vi "hydraharp_acquire_fast.vi"(8 "error in (no error)":errorcluster, 10 "hydraharp_panel out":refnum<class "hydraharp_panel.lvclass">, 11 "hydraharp in":refnum<class "hydraharp.lvclass">) -> (0 "error out":errorcluster, 3 "hydraharp out":refnum<class "hydraharp.lvclass">)   [LabVIEW 2015, in "hydraharp.lvclass"]
uses:
  hydraharp.lvclass
  record_type.ctl
  hydraharp_panel/hydraharp_panel.lvclass
  hydraharp.lvclass/hydraharp.ctl
  UI/panel_class/panel.lvclass/panel.ctl
  hydraharp_fifo_queue_data.ctl
  hydraharp_fifo_actions.ctl
  UI/panel_class/panel.lvclass
panel:
  out "Log Type":T1
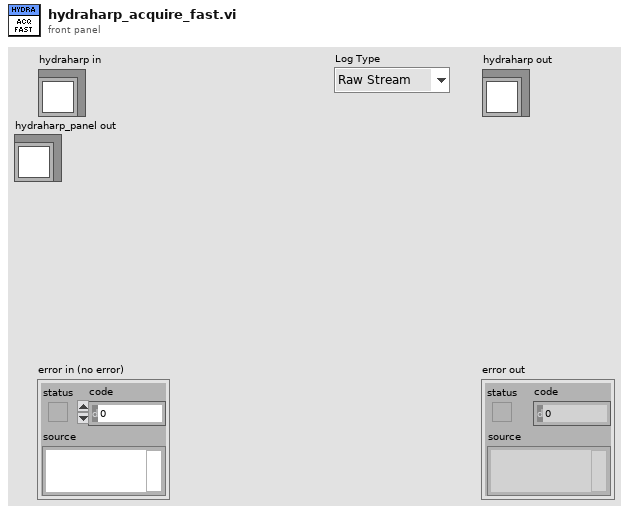
[diagram p1: front panel]
types:
  T1 = typedef "record_type.ctl" = enum16{"Raw Stream", "Processed Records (hdf5)"}
  T2 = typedef "hydraharp_fifo_queue_data.ctl" = cluster{"fifo_buffer":u32[], "fifo_action":T3}
  T3 = typedef "hydraharp_fifo_actions.ctl" = enum16{"stop", "new_data"}
  T4 = typedef "ui_user_events.ctl" = cluster{"update_xy_graph":refnum<user-event>, "update_graph":refnum<user-event>, "update_chart":refnum<user-event>, "update_map":refnum<user-event>, "event_loop_stop":refnum<user-event>, "keep_map":refnum<user-event>}
  T5 = cluster{"log_bin_edges":dbl[], "ch1_photons":dbl[], "ch2_photons":dbl[], "elements_in_record_buffers":i32[], "number_of_new_photons":i32[]}
  T6 = cluster{"stop_fifo_stream":refnum<event-registration>, "Event Registration Refnum":refnum<event-registration>}
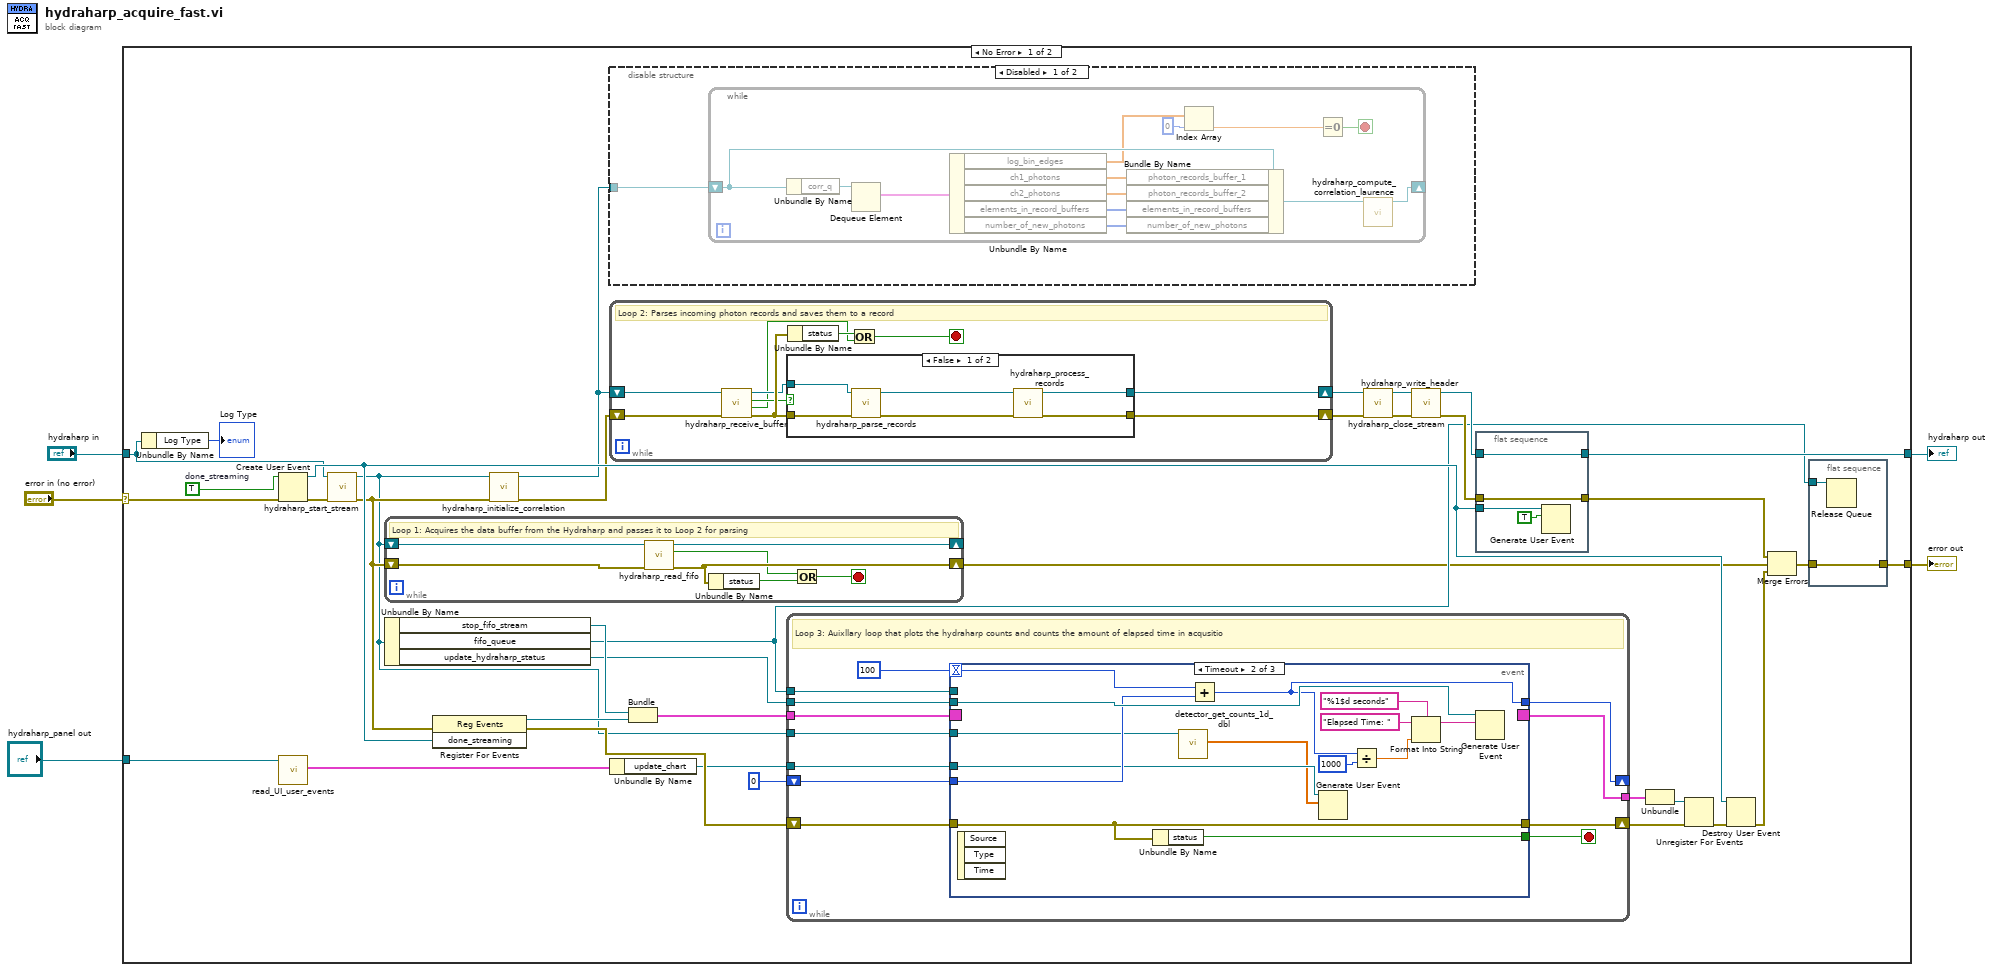
[diagram p0: block diagram]
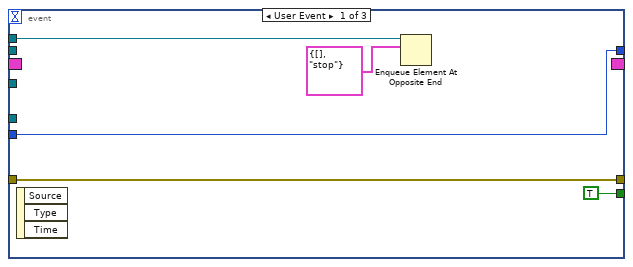
[diagram p3: hidden frame]
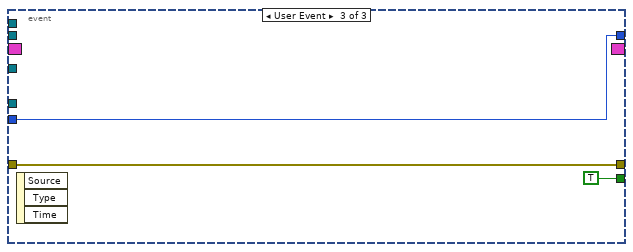
[diagram p4: hidden frame]
diagram:
  n1 = case shown="No Error" "error in (no error)" {
    selector: "error in (no error)" -> [w41 w122]
    tunnel: [w40 w122] -> w4
    tunnel: [w39 w121] -> w3
    tunnel: "hydraharp in" -> [w21 w121]
    tunnel: "hydraharp_panel out" -> [w13 _]
    frame No Error {
      w37 = TRUE  # done_streaming
      n2 = Unbundle By Name(w21) -> ("Log Type"=→"Log Type":T1)
      n3 = Create User Event(user event datatype=w37, error in=w41) -> (user event=w26:refnum<user-event>, error out=w35:errorcluster)
      n4 = call "read_UI_user_events.vi"("panel in"=w13) -> ("ui_user_events"=w12:T4)  [unwired: 8 in, 2 out]
      n5 = call "hydraharp_start_stream.vi"("error in (no error)"=w35, "hydraharp in"=w21) -> ("error out"=w18:errorcluster, "hydraharp out"=w14:refnum<class "hydraharp.lvclass">)  [unwired: 8 in]
      n6 = while {
        shift-right: [w99] -> _
        shift-left: w14 -> [w102]
        shift-right: [w100] -> w10
        shift-left: w18 -> [w101]
        stop <- w98 stop-if-true
        # "Loop 1: Acquires the data buffer from the Hydraharp and passes it to Loop 2 for parsing"
        n7 = call "hydraharp_read_fifo.vi"("error in (no error)"=w101, "hydraharp in"=w102) -> ("error out"=w100:errorcluster, "stop"=w96:bool, "hydraharp out"=w99:refnum<class "hydraharp.lvclass">)  [unwired: 7 in]
        n8 = Unbundle By Name(w100) -> ("status"=w97:bool)
        n9 = Or(x=w96, y=w97) -> (x .or. y?=w98:bool)
      }
      n10 = Unbundle By Name(w14) -> ("stop_fifo_stream"=w34:refnum<event-registration>, "fifo_queue"=w22:refnum<queue>, "update_hydraharp_status"=w16:refnum<user-event>)
      n11 = register-events(error in=w18, w26) -> (reference out=w33:refnum<event-registration>, error out=w36:errorcluster)  [unwired: 1 in]
      n12 = call "hydraharp_initialize_correlation.vi"("error in (no error)"=w18, "hydraharp in"=w14) -> ("error out"=w17:errorcluster, "hydraharp out"=w19:refnum<class "hydraharp.lvclass">)  [unwired: 8 in]
      n13 = disable-structure shown="Disabled" {
        disable-tunnel: w19 -> [w42 _]
        frame Disabled {
          n14 = while {
            shift-right: [w47] -> _
            shift-left: w42 -> [w54]
            stop <- w46 stop-if-true
            n15 = Unbundle By Name(w54) -> ("corr_q"=w55:refnum<queue>)
            n16 = Dequeue Element(queue=w55) -> (element=w53:T5)  [unwired: 2 in, 3 out]
            n17 = Unbundle By Name(w53) -> ("log_bin_edges"=w45:dbl[], "ch1_photons"=w52:dbl[], "ch2_photons"=w51:dbl[], "elements_in_record_buffers"=w50:i32[], "number_of_new_photons"=w49:i32[])
            n18 = Bundle By Name(cluster=w54, "photon_records_buffer_1"=w52, "photon_records_buffer_2"=w51, "elements_in_record_buffers"=w50, "number_of_new_photons"=w49) -> (w48:refnum<class "hydraharp.lvclass">)
            n19 = Index Array(array=w45, index=0) -> (element=w43:dbl)
            n20 = Equal To 0?(x=w43) -> (x = 0?=w46:bool)
            n21 = call "hydraharp_compute_correlation_laurence.vi"("hydraharp in"=w48) -> ("hydraharp out"=w47:refnum<class "hydraharp.lvclass">)  [unwired: 9 in, 1 out]
          }
        }
        frame Enabled {
        }
      }
      n22 = while {
        shift-right: [w106] -> w7
        shift-left: w19 -> [w111]
        shift-right: [w105] -> w9
        shift-left: w17 -> [w112]
        stop <- w109 stop-if-true
        # "Loop 2: Parses incoming photon records and saves them to a record"
        n23 = call "hydraharp_receive_buffer.vi"("error in (no error)"=w112, "hydraharp in"=w111) -> ("error out"=w108:errorcluster, "stop"=w103:bool, "queue_timed_out"=w104:bool, "hydraharp out"=w107:refnum<class "hydraharp.lvclass">)  [unwired: 6 in]
        n24 = case shown="False" w104 {
          tunnel: w108 -> [w117 w120]
          tunnel: w107 -> [w118 w119]
          tunnel: [w114 w119] -> w106
          tunnel: [w113 w120] -> w105
          frame False {
            n25 = call "hydraharp_parse_records.vi"("error in (no error)"=w117, "hydraharp in"=w118) -> ("error out"=w116:errorcluster, "hydraharp out"=w115:refnum<class "hydraharp.lvclass">)  [unwired: 8 in]
            n26 = call "hydraharp_process_records.vi"("error in (no error)"=w116, "hydraharp in"=w115) -> ("error out"=w113:errorcluster, "hydraharp out"=w114:refnum<class "hydraharp.lvclass">)  [unwired: 8 in]
          }
          frame True {
          }
        }
        n27 = Unbundle By Name(w108) -> ("status"=w110:bool)
        n28 = Or(x=w110, y=w103) -> (x .or. y?=w109:bool)
      }
      n29 = Unbundle By Name(w12) -> ("update_chart"=w11:refnum<user-event>)
      n30 = Bundle("stop_fifo_stream"=w34, "Event Registration Refnum"=w33) -> (w32:T6)  [unwired: 1 in]
      n31 = while {
        tunnel: w22 -> [w72]
        tunnel: [w71] -> w31
        shift-right: [w68] -> w38
        shift-left: w36 -> [w69]
        tunnel: w32 -> [w67]
        tunnel: w16 -> [w66]
        shift-right: [w64] -> _
        shift-left: 0 -> [w65]
        tunnel: w14 -> [w63]
        tunnel: w11 -> [w62]
        stop <- w73 stop-if-true
        # "Loop 3: Auixllary loop that plots the hydraharp counts and counts the amount of elapsed time in acqusitio"
        n32 = event shown="[1] Timeout" {
          selector: w67 -> [_ _ _]
          dyn-events: [_ _ _] -> w71
          timeout: 100 -> [_ w88 _]
          tunnel: [TRUE w92 TRUE] -> w73
          tunnel: w72 -> [w77 _ _]
          tunnel: w69 -> [w75 w91 w94]
          tunnel: [w75 w91 w94] -> w68
          tunnel: w66 -> [_ w90 _]
          tunnel: w65 -> [w74 w87 w93]
          tunnel: [w74 w82 w93] -> w64
          tunnel: w63 -> [_ w81 _]
          tunnel: w62 -> [_ w80 _]
          event User Event {
            n33 = event-data() -> ()  [unwired: 1 in, 3 out]
            n34 = Enqueue Element At Opposite End(queue=w77, element=T2 {"fifo_buffer"=[], "fifo_action"=enum."stop"}) -> ()  [unwired: 2 in, 3 out]
          }
          event Timeout {
            n35 = event-data() -> ()  [unwired: 1 in, 3 out]
            n36 = Unbundle By Name(w91) -> ("status"=w92:bool)
            n37 = call-dynamic "detector_get_counts_1d_dbl.vi"("hydraharp in"=w81) -> ("counts"=w79:dbl[])  [unwired: 8 in, 2 out]
            n38 = Add(x=w88, y=w87) -> (x+y=w82:i32)
            n39 = Generate User Event(user event=w80, event data cluster=w79) -> ()  [unwired: 2 in, 2 out]
            n40 = Divide(x=w82, y=1000) -> (x/y=w84:dbl)
            n41 = Format Into String(format string="%1$d seconds", initial string="Elapsed Time: ", w84) -> (resulting string=w83:string)  [unwired: 1 in, 1 out]
            n42 = Generate User Event(user event=w90, event data cluster=w83) -> ()  [unwired: 2 in, 2 out]
          }
          event User Event {
            n43 = event-data() -> ()  [unwired: 1 in, 3 out]
          }
        }
      }
      n44 = call "hydraharp_write_header.vi"("error in (no error)"=w9, "hydraharp in"=w7) -> ("error out"=w8:errorcluster, "hydraharp out"=w6:refnum<class "hydraharp.lvclass">)  [unwired: 8 in]
      n45 = call "hydraharp_close_stream.vi"("error in (no error)"=w8, "hydraharp in"=w6) -> ("error out"=w28:errorcluster, "hydraharp out"=w27:refnum<class "hydraharp.lvclass">)  [unwired: 8 in]
      n46 = flat-sequence {
        tunnel: w28 -> [w58]
        tunnel: w27 -> [w61]
        tunnel: [w61] -> w39
        tunnel: w26 -> [w60]
        tunnel: [w58] -> w25
        frame #0 {
          n47 = Generate User Event(user event=w60, event data cluster=TRUE ("event data")) -> ()  [unwired: 2 in, 2 out]
        }
      }
      n48 = Unbundle(w31) -> ("Event Registration Refnum"=w30:refnum<event-registration>)  [unwired: 1 out]
      n49 = Unregister For Events(event registration refnum=w30, error in=w38) -> (error out=w24:errorcluster)
      n50 = Destroy User Event(user event=w26, error in=w24) -> (error out=w29:errorcluster)
      n51 = Merge Errors(w25, w10, w29) -> (w23:errorcluster)
      n52 = flat-sequence {
        tunnel: w23 -> [w56]
        tunnel: w22 -> [w57]
        tunnel: [w56] -> w40
        frame #0 {
          n53 = Release Queue(queue=w57) -> ()  [unwired: 2 in, 3 out]
        }
      }
    }
    frame Error {
    }
  }
  "error out" <- w4
  "hydraharp out" <- w3
